vi "authority_variable.vi"(2 "Authority_In":u16(ring) items=["学生", "老师"], 3 "select":enum16{"Read", "Write"}(ring)) -> (1 "Authority_Out":u16)   [LabVIEW 2015]
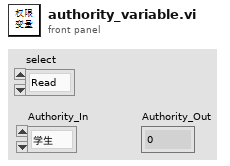
[diagram p1: front panel]
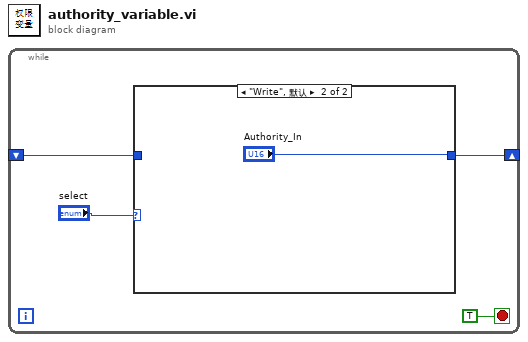
[diagram p0: block diagram]
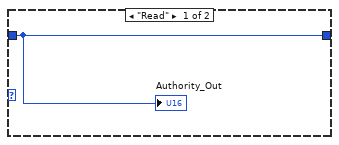
[diagram p2: hidden frame]
diagram:
  n1 = while {
    shift-right: [w2] -> _
    shift-left: _ -> [w1]
    stop <- TRUE stop-if-true
    n2 = case shown="\"Write\", 默认" "select" {
      tunnel: [w5 "Authority_In"] -> w2
      tunnel: w1 -> [w5 _]
      frame "Read" {
        "Authority_Out" <- w5
      }
      frame "Write", Default {
      }
    }
  }
